vi "Get Array Element Offsets.vi"(8 "error in (no error)":errorcluster, 10 "Offset":i32, 11 "JSON":string) -> (0 "error out":errorcluster, 1 "Elements":T2(array[cluster]), 2 "Offset past Array":i32)   [LabVIEW 2013, in "JSONtext.lvlib"]
uses:
  JSONtext.lvlib
  Parsing State.ctl
  Advance past String.vi
  Advance past Number.vi
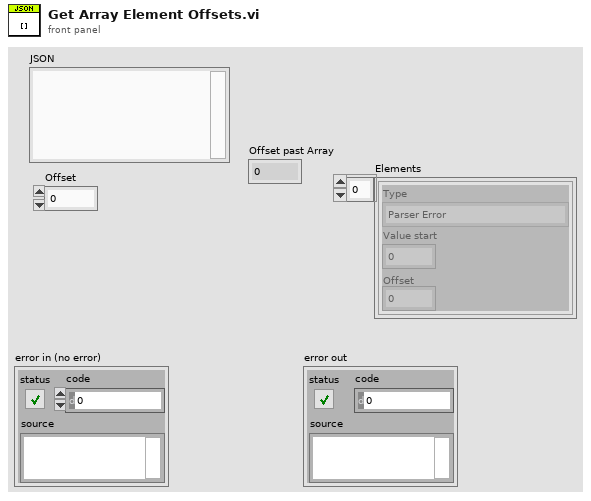
[diagram p1: front panel]
types:
  T1 = typedef "JSONtext.lvlib/Parsing State.ctl" = enum16{"Parser Error", "Object", "Array", "String", "Number/Other", "Leading Whitespace", "Object end", "Array end", "Value end"}
  T2 = cluster{"Type":T1, "Value start":i32, "Offset":i32}[]
  T3 = cluster{"Type":T1, "Value start":i32, "Offset":i32}
  T4 = cluster{"State":T1, "Value start":i32, "index":i32}
  T5 = cluster{"State":T1, "Value start":i32, "index":i32}[]
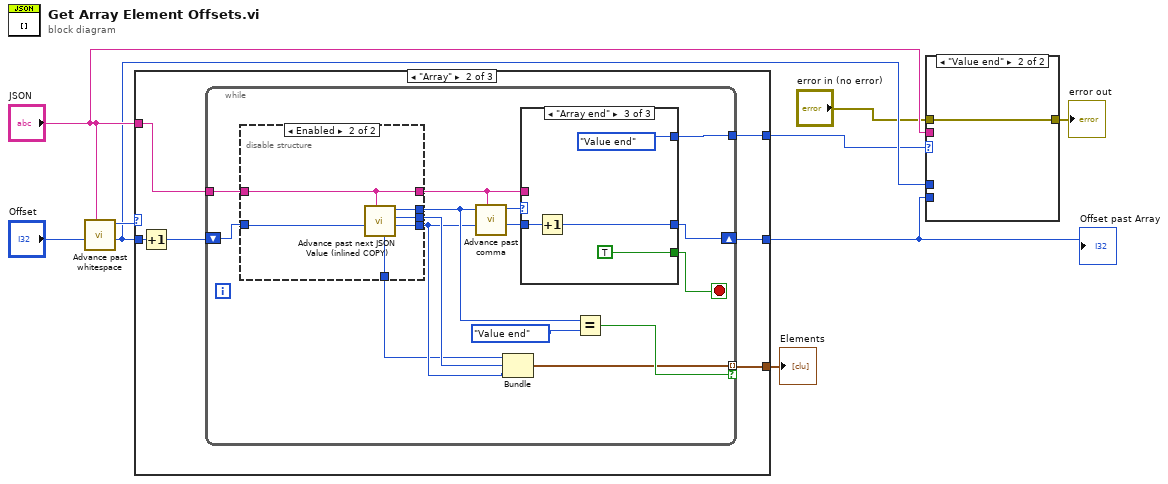
[diagram p0: block diagram]
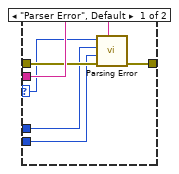
[diagram p2: hidden frame]
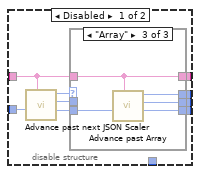
[diagram p4: hidden frame]
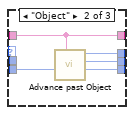
[diagram p6: hidden frame]
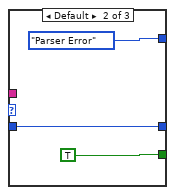
[diagram p8: hidden frame]
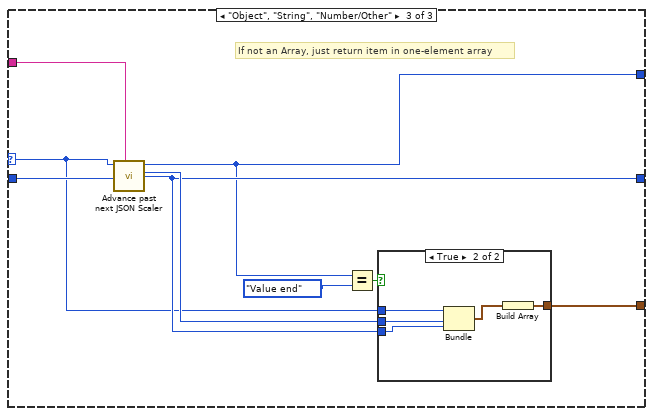
[diagram p9: hidden frame]
diagram:
  n1 = call "Advance past whitespace.vi"("JSON"="JSON", "Offset"="Offset") -> ("Offset of first non-whitespace"=w6:i32, "State"=w8:T1)  [unwired: 8 in]
  n2 = case shown="\"Array\"" w8 {
    selector: w8 -> [w11 _ w71]
    tunnel: [w11 w17 w73] -> w2
    tunnel: [w10 w16 w75] -> w5
    tunnel: [_ w14 w70] -> w1
    tunnel: "JSON" -> [_ w13 w74]
    tunnel: w6 -> [w10 w12 w78]
    frame "Parser Error", Default {
    }
    frame "Array" {
      n3 = Increment(x=w12) -> (x+1=w15:i32)
      n4 = while {
        tunnel: w13 -> [w26]
        shift-right: [w29] -> w16
        shift-left: w15 -> [w30]
        tunnel: [w27] -> w17
        tunnel: [w18] -> w14 mode=indexing if=w22
        stop <- w28 stop-if-true
        n5 = disable-structure shown="Enabled" {
          disable-tunnel: w30 -> [w41 w58]
          disable-tunnel: w26 -> [w38 w57]
          disable-tunnel: [w37 w60] -> w21
          disable-tunnel: [w36 w61] -> w20
          disable-tunnel: [w35 w57] -> w25
          disable-tunnel: [w33 w59] -> w23
          disable-tunnel: [_ w56] -> w19
          frame Disabled {
            n6 = call "Advance past next JSON Scaler.vi"("JSON"=w38, "Offset"=w41) -> ("index"=w39:i32, "Value start"=w34:i32, "Enum"=w40:T1)  [unwired: 7 in]
            n7 = case shown="\"Array\"" w40 {
              selector: w40 -> [w44 _ _]
              tunnel: w39 -> [w43 w50 w51]
              tunnel: [w44 w49 w54] -> w33
              tunnel: [w43 w48 w55] -> w36
              tunnel: w38 -> [w45 w47 w53]
              tunnel: [w45 w47 w53] -> w35
              tunnel: [w42 w46 w52] -> w37
              tunnel: w34 -> [w42 _ _]
              frame Default {
              }
              frame "Object" {
                n8 = call "Advance past Object.vi"("JSON"=w47, "Offset"=w50) -> ("Offset past Object"=w48:i32, "Object Start"=w46:i32, "State"=w49:T1)  [unwired: 7 in]
              }
              frame "Array" {
                n9 = call "Advance past Array.vi"("JSON"=w53, "Offset"=w51) -> ("Offset past match"=w55:i32, "Start"=w52:i32, "State"=w54:T1)  [unwired: 7 in]
              }
            }
          }
          frame Enabled {
            n10 = call "Advance past next JSON Value (inlined COPY).vi"("JSON"=w57, "Offset"=w58) -> ("Offset"=w61:i32, "Value start"=w60:i32, "State"=w59:T1, "Type"=w56:T1)  [unwired: 6 in]
          }
        }
        n11 = call "Advance past comma.vi"("JSON"=w25, "Offset"=w20, "State in"=w23) -> ("Offset past match"=w32:i32, "State"=w31:T1)  [unwired: 7 in]
        n12 = Bundle("Type"=w19, "Value start"=w21, "Offset"=w20) -> (w18:T3)  [unwired: 1 in]
        n13 = case shown="\"Array end\"" w31 {
          tunnel: [_ TRUE TRUE] -> w28
          tunnel: [_ Parsing_State."Parser Error" Parsing_State."Value end"] -> w27
          tunnel: w32 -> [w62 w63 w67]
          tunnel: [w62 w63 w66] -> w29
          tunnel: w25 -> [_ _ _]
          frame "Leading Whitespace" {
          }
          frame Default {
          }
          frame "Array end" {
            n14 = Increment(x=w67) -> (x+1=w66:i32)
          }
        }
        n15 = Equal?(x=w23, y=Parsing_State."Value end") -> (x = y?=w22:bool)
      }
    }
    frame "Object", "String", "Number/Other" {
      # "If not an Array, just return item in one-element array"
      n16 = call "Advance past next JSON Scaler.vi"("JSON"=w74, "Offset"=w78, "State"=w71) -> ("index"=w75:i32, "Value start"=w76:i32, "Enum"=w73:T1)  [unwired: 6 in]
      n17 = Equal?(x=w73, y=Parsing_State."Value end") -> (x = y?=w72:bool)
      n18 = case shown="True" w72 {
        tunnel: w76 -> [_ w81]
        tunnel: w75 -> [_ w82]
        tunnel: [_ w83] -> w70
        tunnel: w71 -> [_ w80]
        frame False {
        }
        frame True {
          n19 = Bundle("State"=w80, "Value start"=w81, "index"=w82) -> (w79:T4)  [unwired: 1 in]
          n20 = Build Array(w79) -> (w83:T5)
        }
      }
    }
  }
  "Offset past Array" <- w5
  "Elements" <- w1
  n21 = case shown="\"Value end\"" w2 {
    selector: w2 -> [w84 _]
    tunnel: "JSON" -> [w89 _]
    tunnel: "error in (no error)" -> [w88 w90]
    tunnel: [w87 w90] -> w4
    tunnel: w6 -> [w86 _]
    tunnel: w5 -> [w85 _]
    frame "Parser Error", Default {
      n22 = call "Parsing Error.vi"("JSON"=w89, "error in (no error)"=w88, "Offset past match"=w85, "Value start"=w86, "State"=w84) -> ("error out"=w87:errorcluster)  [unwired: 6 in]
    }
    frame "Value end" {
    }
  }
  "error out" <- w4
